vi "Plot Format 2D Table.vi"(8 "Data 2D Table":cluster{"X":sgl[], "Y":sgl[], "Z":sgl[][]}, 11 "Table Ref":refnum<vi>) -> ()   [LabVIEW 2016]
uses:
  <vilib>/Utility/miscctls.llb/LVRowAndColumnTypeDef.ctl
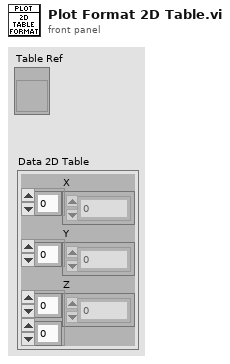
[diagram p1: front panel]
types:
  T1 = typedef "LVRowAndColumnTypeDef.ctl" = cluster{"Row":i32, "Column":i32}
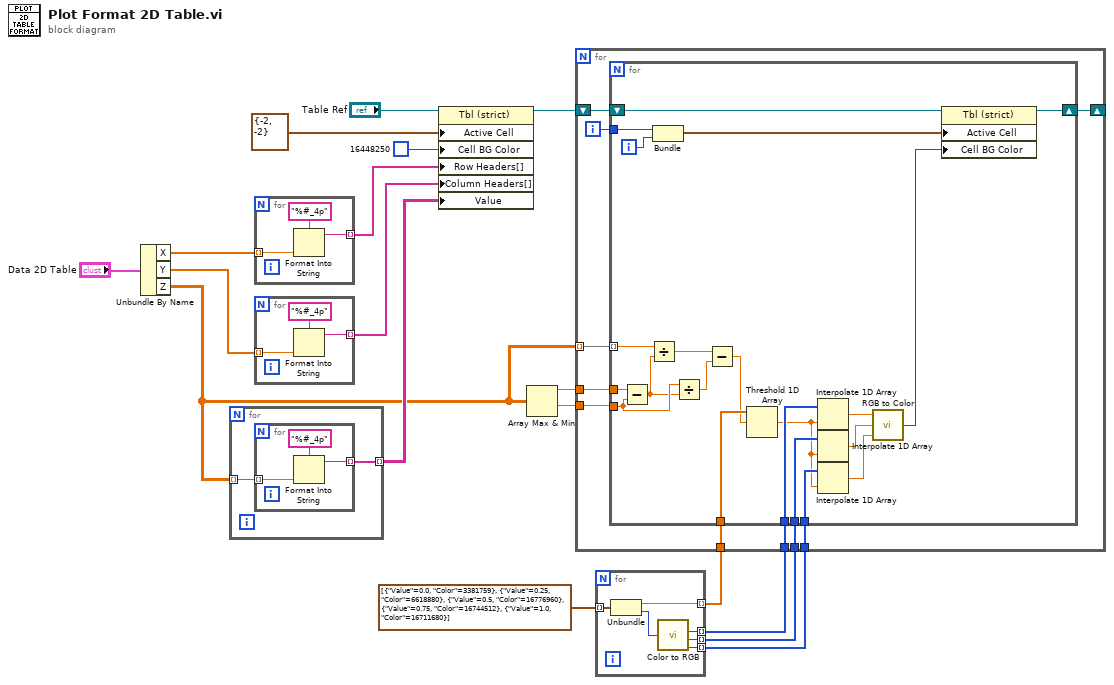
[diagram p0: block diagram]
diagram:
  n1 = Unbundle By Name("Data 2D Table") -> ("X"=w17:sgl[], "Y"=w16:sgl[], "Z"=w10:sgl[][])
  n2 = for {
    tunnel: w10 -> [w20] mode=indexing
    tunnel: [w19] -> w13 mode=indexing
    n3 = for {
      tunnel: w20 -> [w23] mode=indexing
      tunnel: [w21] -> w19 mode=indexing
      n4 = Format Into String(format string="%#_4p", w23) -> (resulting string=w21:string)  [unwired: 2 in, 1 out]
    }
  }
  n5 = for {
    tunnel: w17 -> [w26] mode=indexing
    tunnel: [w24] -> w15 mode=indexing
    n6 = Format Into String(format string="%#_4p", w26) -> (resulting string=w24:string)  [unwired: 2 in, 1 out]
  }
  n7 = for {
    tunnel: w16 -> [w29] mode=indexing
    tunnel: [w27] -> w14 mode=indexing
    n8 = Format Into String(format string="%#_4p", w29) -> (resulting string=w27:string)  [unwired: 2 in, 1 out]
  }
  n9 = property on="Property Node" class="Tbl (strict)"(reference="Table Ref", "Active Cell"=T1 {"Row"=-2, "Column"=-2} ("Active Cell:Active Cell"), "Cell BG Color"=u32 16448250 ("Active Cell:Cell Background Color"), "Row Headers[]"=w15, "Column Headers[]"=w14, "Value"=w13) -> (reference out=w9:refnum<vi>)  [unwired: 1 in, 1 out]
  n10 = Array Max & Min(array=w10) -> (max value=w12:sgl, min value=w11:sgl)  [unwired: 2 out]
  n11 = for {
    tunnel: cluster{"Value":sgl, "Color":u32}[] [{"Value"=0.0, "Color"=3381759}, {"Value"=0.25, "Color"=6618880}, {"Value"=0.5, "Color"=16776960}, {"Value"=0.75, "Color"=16744512}, {"Value"=1.0, "Color"=16711680}] -> [w35] mode=indexing
    tunnel: [w33] -> w7 mode=indexing
    tunnel: [w32] -> w6 mode=indexing
    tunnel: [w31] -> w5 mode=indexing
    tunnel: [w30] -> w4 mode=indexing
    n12 = Unbundle(w35) -> ("Value"=w30:sgl, "Color"=w34:u32)
    n13 = call <vilib>:"Color to RGB.vi"("Color"=w34) -> ("R"=w33:u8, "G"=w32:u8, "B"=w31:u8)  [unwired: 1 out]
  }
  n14 = for {
    tunnel: w12 -> [w45]
    tunnel: w11 -> [w44]
    tunnel: w10 -> [w43] mode=indexing
    shift-right: [w40] -> _
    shift-left: w9 -> [w41]
    tunnel: w7 -> [w39]
    tunnel: w6 -> [w38]
    tunnel: w5 -> [w37]
    tunnel: w4 -> [w36]
    i -> [w42]
    n15 = for {
      tunnel: w43 -> [w66] mode=indexing
      tunnel: w45 -> [w65]
      tunnel: w44 -> [w64]
      tunnel: w42 -> [w57]
      shift-right: [w52] -> w40
      shift-left: w41 -> [w54]
      tunnel: w39 -> [w51]
      tunnel: w38 -> [w50]
      tunnel: w37 -> [w49]
      tunnel: w36 -> [w48]
      i -> [w56]
      n16 = Subtract(x=w65, y=w64) -> (x-y=w63:sgl)
      n17 = Divide(x=w66, y=w63) -> (x/y=w62:sgl)
      n18 = Bundle(w57, w56) -> (w55:cluster{i32, i32})  [unwired: 1 in]
      n19 = Divide(x=w64, y=w63) -> (x/y=w61:sgl)
      n20 = Subtract(x=w62, y=w61) -> (x-y=w46:sgl)
      n21 = Threshold 1D Array(2:w46, 3:w48) -> (0:w47:sgl)  [unwired: 1 in]
      n22 = Interpolate 1D Array(1:w47, 2:w51) -> (0:w58:dbl)
      n23 = Interpolate 1D Array(1:w47, 2:w50) -> (0:w59:dbl)
      n24 = Interpolate 1D Array(1:w47, 2:w49) -> (0:w60:dbl)
      n25 = call <vilib>:"RGB to Color.vi"("B"=w60, "G"=w59, "R"=w58) -> ("Color"=w53:u32)
      n26 = property on="Property Node" class="Tbl (strict)"(reference=w54, "Active Cell"=w55, "Cell BG Color"=w53) -> (reference out=w52:refnum<vi>)  [unwired: 1 in, 1 out]
    }
  }
